vi "Build SCPI Command.vi"(8 "error in":errorcluster, 9 "Noun(s)":string, 10 "Verb":T4, 11 "Mercury Reference In":T1) -> (0 "error out":errorcluster, 2 "SCPI Message(s)":string[](array[string]), 3 "Mercury Reference Out":T1)   [LabVIEW 2015, in "Mercury iXX.lvlib"]
uses:
  Mercury iXX.lvlib
  Controls/Command Verbs.ctl
  Public/Controls/Mercury Reference.ctl
  Public/Controls/Comms Transport Layer.ctl
  Controls/Query Dynamic Reference.ctl
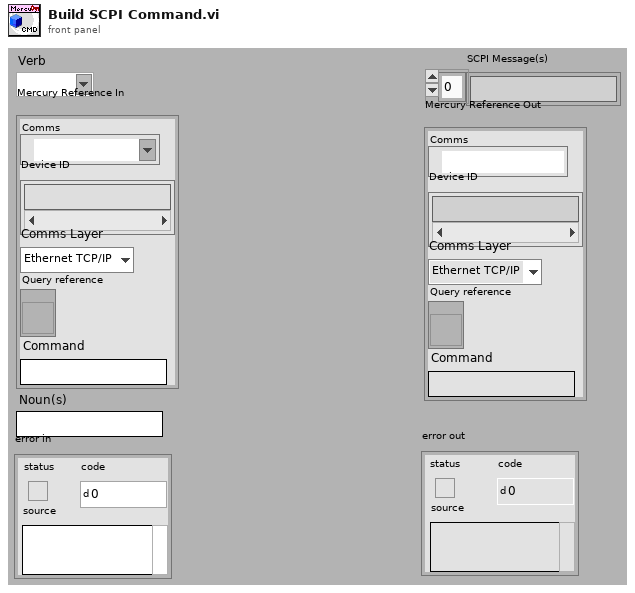
[diagram p1: front panel]
types:
  T1 = typedef "Mercury iXX.lvlib/Mercury Reference.ctl" = cluster{"Comms":refnum<visa-resource-name>, "Device ID":string[], "Comms Layer":T2, "Command":string, "Query reference":T3}
  T2 = typedef "Mercury iXX.lvlib/Comms Transport Layer.ctl" = enum16{"Ethernet TCP/IP", "USB", "ISOBus - RS-232", "GPIB"}
  T3 = typedef "Mercury iXX.lvlib/Query Dynamic Reference.ctl" = refnum<vi>
  T4 = typedef "Mercury iXX.lvlib/Command Verbs.ctl" = string
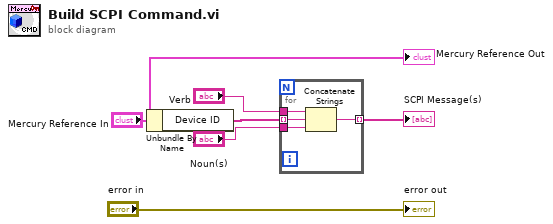
[diagram p0: block diagram]
diagram:
  n1 = Unbundle By Name("Mercury Reference In") -> ("Device ID"=w3:string[])
  n2 = for {
    tunnel: "Verb" -> [w10]
    tunnel: "Noun(s)" -> [w8]
    tunnel: w3 -> [w9] mode=indexing
    tunnel: [w7] -> w6 mode=indexing
    n3 = Concatenate Strings(w10, w9, w8) -> (w7:string)
  }
  "SCPI Message(s)" <- w6
  "error out" <- "error in"
  "Mercury Reference Out" <- "Mercury Reference In"
